vi "Facade.vi"(0 "Data In":T5, 2 "Display State In":T2={"Pause"=FALSE, "Camera"={"Position"={"X"=0.0, "Y"=0.0, "Z"=4.0}, "Target"={"X"=0.0, "Y"=0.0, "Z"=0.0}, "Up Direction"={"X"=0.0, "Y"=1.0, "Z"=0.0}}, "Background Color"={"Red"=0.0, "Green"=0.0, "Blue"=0.0, "Alpha"=0.0}, "3DRefnum"=refnum}, 3 "Container State":T4) -> (6 "Data Out":T5, 7 "Display State Out":T2={"Pause"=FALSE, "Camera"={"Position"={"X"=0.0, "Y"=0.0, "Z"=4.0}, "Target"={"X"=0.0, "Y"=0.0, "Z"=0.0}, "Up Direction"={"X"=0.0, "Y"=1.0, "Z"=0.0}}, "Background Color"={"Red"=0.0, "Green"=0.0, "Blue"=0.0, "Alpha"=0.0}, "3DRefnum"=refnum}, 8 "Action":T1)   [LabVIEW 2017, in "Simulator Display.xctl"]
uses:
  <vilib>/robotics/Controls/Simulator Display/Simulator Display.xctl
  <vilib>/robotics/Controls/Simulator Display/Data.ctl
  <vilib>/_xctls/Container State.ctl
  <vilib>/robotics/Controls/Simulator Display/State.ctl
  <vilib>/Utility/miscctls.llb/LVRGBAColorTypeDef.ctl
  <vilib>/_xctls/Action.ctl
  <vilib>/_xctls/XControlSupport.lvlib
panel:
  out "3D Picture":refnum<vi>(3d-picture)
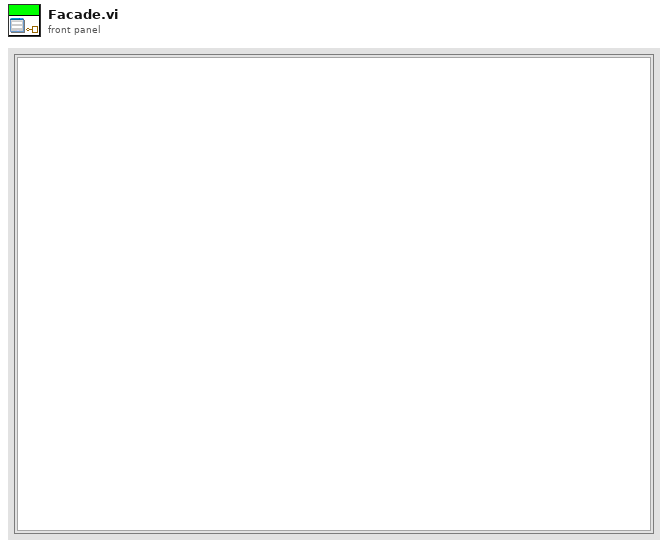
[diagram p1: front panel]
types:
  T1 = typedef "XControlSupport.lvlib/Action.ctl" = cluster{"Data Changed?":bool, "State Changed?":bool, "Action Name":string}
  T2 = typedef "Simulator Display.xctl/State.ctl" = cluster{"Pause":bool, "Camera":cluster{"Position":cluster{"X":dbl, "Y":dbl, "Z":dbl}, "Target":cluster{"X":dbl, "Y":dbl, "Z":dbl}, "Up Direction":cluster{"X":dbl, "Y":dbl, "Z":dbl}}, "Background Color":T3, "3DRefnum":refnum<vi>}
  T3 = typedef "LVRGBAColorTypeDef.ctl" = cluster{"Red":sgl, "Green":sgl, "Blue":sgl, "Alpha":sgl}
  T4 = typedef "XControlSupport.lvlib/Container State.ctl" = cluster{"Indicator?":bool, "Run Mode?":bool, " Refnum":refnum<vi>}
  T5 = typedef "Simulator Display.xctl/Data.ctl" = refnum<vi>
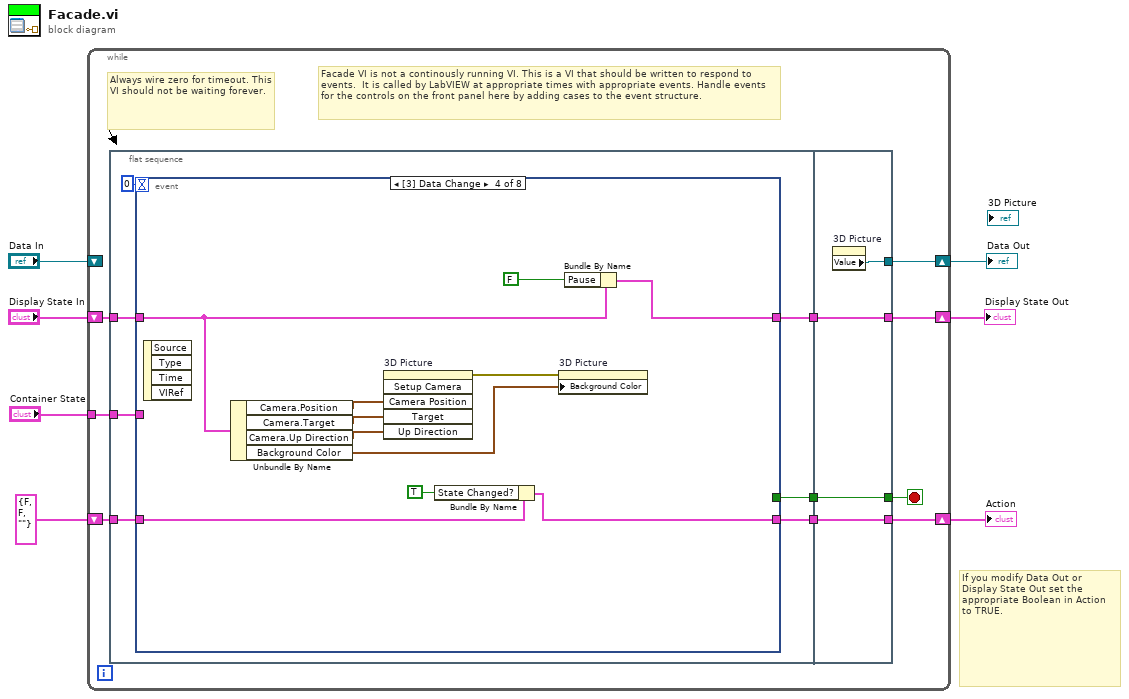
[diagram p0: block diagram]
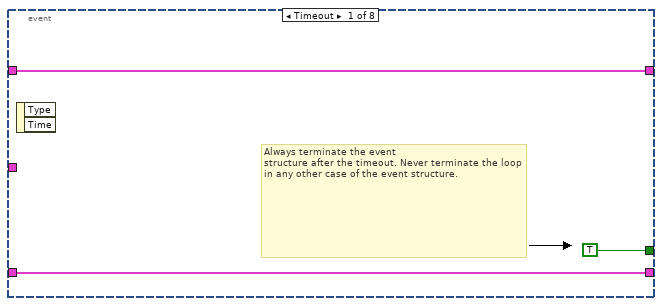
[diagram p2: hidden frame]
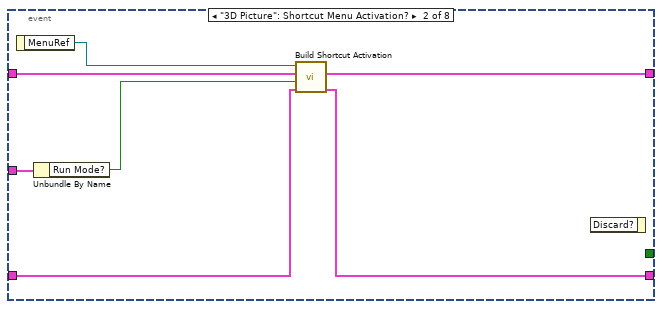
[diagram p3: hidden frame]
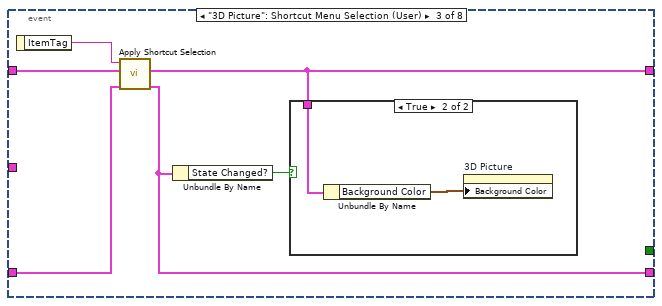
[diagram p4: hidden frame]
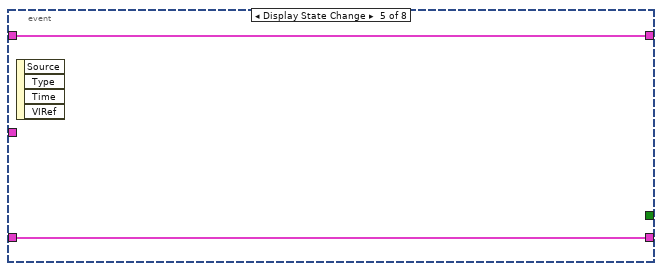
[diagram p6: hidden frame]
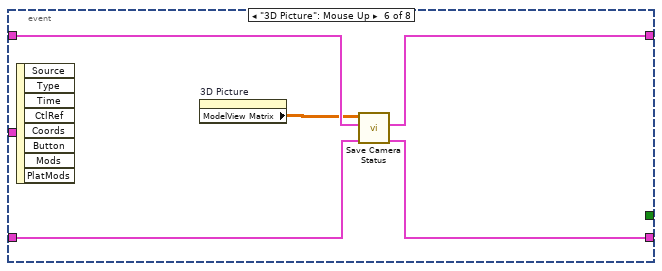
[diagram p7: hidden frame]
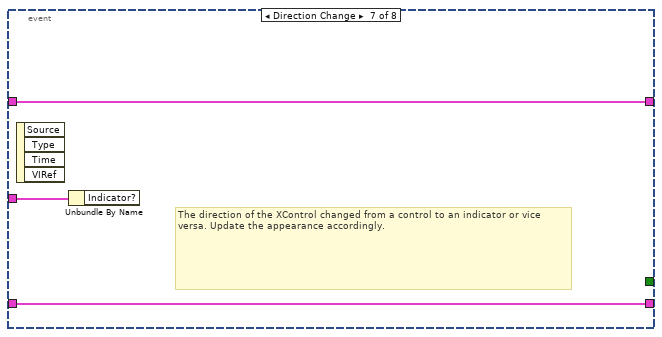
[diagram p8: hidden frame]
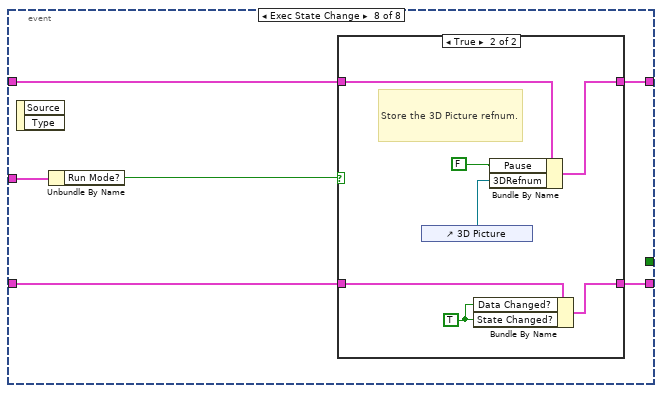
[diagram p9: hidden frame]
diagram:
  # "If you modify Data Out or\nDisplay State Out set the\nappropriate Boolean in Action\nto TRUE."
  n1 = while {
    shift-right: [w16] -> w6
    shift-left: "Display State In" -> [w17]
    tunnel: "Container State" -> [w14]
    shift-right: [w12] -> w4
    shift-left: T1 {"Data Changed?"=FALSE, "State Changed?"=FALSE, "Action Name"=""} ("Action") -> [w13]
    shift-right: [w8] -> w1
    shift-left: "Data In" -> [_]
    stop <- w15 stop-if-true
    # "Facade VI is not a continously running VI. This is a VI that should be written to respond to events.  It is called by LabVIEW at appropriate times with appropriate events. Handle events for the controls on the front panel here by adding cases to the event structure."
    # "Always wire zero for timeout. This\nVI should not be waiting forever."
    n2 = flat-sequence {
      tunnel: w17 -> [w24]
      tunnel: w14 -> [w20]
      tunnel: w13 -> [w19]
      tunnel: [w23] -> w11
      tunnel: [w22] -> w10
      tunnel: [w18] -> w9
      tunnel: [w80] -> w12
      tunnel: [w81] -> w15
      tunnel: [w82] -> w16
      tunnel: w11 -> [w82]
      tunnel: w10 -> [w81]
      tunnel: w9 -> [w80]
      tunnel: [w79] -> w8
      frame #0 {
        n3 = event shown="[3] Data Change" {
          selector: _ -> [_ _ _ _ _ _ _ _]
          dyn-events: _ -> [_ _ _ _ _ _ _ _]
          timeout: 0 -> [_ _ _ _ _ _ _ _]
          tunnel: w24 -> [w26 w33 w40 w45 w54 w60 w62 w67]
          tunnel: [w26 w30 w35 w44 w54 w59 w62 w66] -> w23
          tunnel: [TRUE _ _ _ _ _ _ _] -> w22
          tunnel: w20 -> [_ w34 _ _ _ _ w63 w69]
          tunnel: [w25 w28 w37 w52 w55 w57 w61 w65] -> w18
          tunnel: w19 -> [w25 w29 w39 w53 w55 w58 w61 w64]
          event Timeout {
            # "Always terminate the event\nstructure after the timeout. Never terminate the loop in any other case of the event structure."
            n4 = event-data() -> ()  [unwired: 1 in, 2 out]
          }
          event "3D Picture": Shortcut Menu Activation? {
            n5 = event-data() -> ("MenuRef"=w32:refnum<k9>)  [unwired: 1 in]
            n6 = Unbundle By Name(w34) -> ("Run Mode?"=w31:bool)
            n7 = call <vilib>:"Build Shortcut Activation.vi"("Action In"=w29, "Run Mode?"=w31, "Display State In"=w33, "MenuRef in"=w32) -> ("Action Out"=w28:T1, "Display State Out"=w30:T2)  [unwired: 5 in, 1 out]
            n8 = event-data() -> ()  [unwired: 2 in, 1 out]
          }
          event "3D Picture": Shortcut Menu Selection (User) {
            n9 = event-data() -> ("ItemTag"=w38:string)  [unwired: 1 in]
            n10 = call <vilib>:"Apply Shortcut Selection.vi"("Action In"=w39, "Display State In"=w40, "ItemTag"=w38) -> ("Action Out"=w37:T1, "Display State Out"=w35:T2)  [unwired: 7 in]
            n11 = Unbundle By Name(w37) -> ("State Changed?"=w36:bool)
            n12 = case shown="True" w36 {
              tunnel: w35 -> [_ w42]
              frame False {
              }
              frame True {
                n13 = Unbundle By Name(w42) -> ("Background Color"=w41:T3)
                n14 = property on="3D Picture" class="SceneGraphDisp (strict)"("Background Color"=w41) -> ()  [unwired: 2 in, 2 out]
              }
            }
          }
          event Data Change {
            n15 = event-data() -> ()  [unwired: 1 in, 4 out]
            n16 = Unbundle By Name(w45) -> ("Camera.Position"=w49:cluster{"X":dbl, "Y":dbl, "Z":dbl}, "Camera.Target"=w48:cluster{"X":dbl, "Y":dbl, "Z":dbl}, "Camera.Up Direction"=w47:cluster{"X":dbl, "Y":dbl, "Z":dbl}, "Background Color"=w50:T3)
            n17 = invoke on="3D Picture" class="SceneGraphDisp (strict)" method="Setup Camera"("Camera Position"=w49, "Target"=w48, "Up Direction"=w47) -> (error out=w46:errorcluster)  [unwired: 3 in, 5 out]
            n18 = Bundle By Name(cluster=w53, "State Changed?"=TRUE ("Data Changed?")) -> (w52:T1)
            n19 = property on="3D Picture" class="SceneGraphDisp (strict)"(error in=w46, "Background Color"=w50) -> ()  [unwired: 1 in, 2 out]
            n20 = Bundle By Name(cluster=w45, "Pause"=FALSE ("Contact Points")) -> (w44:T2)
          }
          event Display State Change {
            n21 = event-data() -> ()  [unwired: 1 in, 4 out]
          }
          event "3D Picture": Mouse Up {
            n22 = event-data() -> ()  [unwired: 1 in, 8 out]
            n23 = property on="3D Picture" class="SceneGraphDisp (strict)"() -> ("ModelView Matrix"=w56:sgl[][])  [unwired: 2 in, 2 out]
            n24 = call <vilib>:"Save Camera Status.vi"("Action In"=w58, "Display State In"=w60, "ModelView Matrix"=w56) -> ("Action Out"=w57:T1, "Display State Out"=w59:T2)  [unwired: 7 in]
          }
          event Direction Change {
            # "The direction of the XControl changed from a control to an indicator or vice versa. Update the appearance accordingly."
            n25 = event-data() -> ()  [unwired: 1 in, 4 out]
            n26 = Unbundle By Name(w63) -> ()  [unwired: 1 out]
          }
          event Exec State Change {
            n27 = event-data() -> ()  [unwired: 1 in, 2 out]
            n28 = Unbundle By Name(w69) -> ("Run Mode?"=w68:bool)
            n29 = case shown="True" w68 {
              tunnel: w67 -> [w71 w78]
              tunnel: [w71 w77] -> w66
              tunnel: w64 -> [w70 w76]
              tunnel: [w70 w75] -> w65
              frame False {
              }
              frame True {
                w73 = TRUE ("State Changed?")
                # "Store the 3D Picture refnum."
                n30 = control-ref of="3D Picture"() -> (w72:refnum<vi>)
                n31 = Bundle By Name(cluster=w76, "Data Changed?"=w73, "State Changed?"=w73) -> (w75:T1)
                n32 = Bundle By Name(cluster=w78, "Pause"=FALSE, "3DRefnum"=w72) -> (w77:T2)
              }
            }
          }
        }
      }
      frame #1 {
        n33 = property on="3D Picture" class="SceneGraphDisp (strict)"() -> ("Value"=w79:refnum<vi>)  [unwired: 2 in, 2 out]
      }
    }
  }
  "Display State Out" <- w6
  "Data Out" <- w1
  "Action" <- w4
